vi "430_RS232_Query.vi"(8 "error in (no error)":errorcluster, 9 "Timeout":i32=1000, 10 "Command":string, 11 "VISA resource name":refnum<visa-resource-name>="COM1") -> (0 "error out":errorcluster, 1 "Bytes Read":i32, 2 "Response":string, 3 "VISA resource name out":refnum<visa-resource-name>="COM1", 4 "Bytes Written":i32)   [LabVIEW 2017]
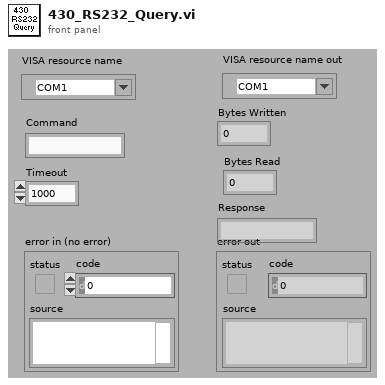
[diagram p1: front panel]
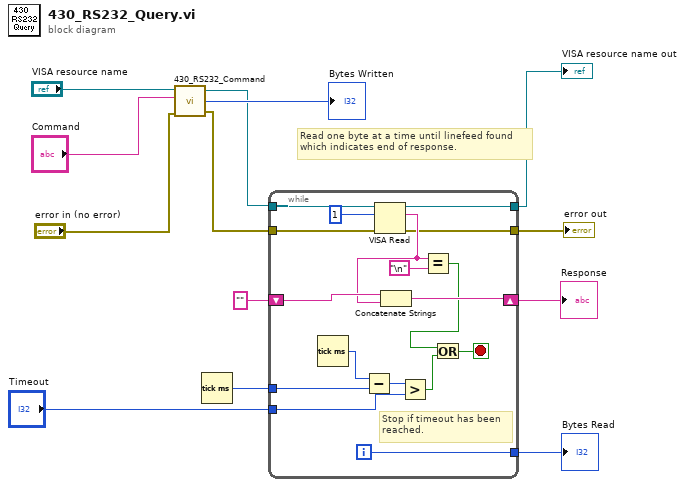
[diagram p0: block diagram]
diagram:
  # "Read one byte at a time until linefeed found\nwhich indicates end of response."
  n1 = call "430_RS232_Command.vi"("error in (no error)"="error in (no error)", "Command"="Command", "VISA resource name"="VISA resource name") -> ("error out"=w7:errorcluster, "bytes written"=→"Bytes Written":i32, "VISA resource name out"=w3:refnum<visa-resource-name>)  [unwired: 1 in]
  n2 = Tick Count (ms)() -> (millisecond timer value=w9:u32)
  n3 = while {
    tunnel: w3 -> [w15]
    tunnel: [w30] -> w4
    tunnel: w7 -> [w29]
    tunnel: [w16] -> w13
    tunnel: [w28] -> w12
    shift-right: [w24] -> w10
    shift-left: "" -> [w26]
    tunnel: "Timeout" -> [w17]
    tunnel: w9 -> [w22]
    i -> [w28]
    stop <- w18 stop-if-true
    # "Stop if timeout has been\nreached."
    n4 = Tick Count (ms)() -> (millisecond timer value=w23:u32)
    n5 = Subtract(x=w23, y=w22) -> (x-y=w21:u32)
    n6 = VISA Read(VISA resource name=w15, byte count=1 ("bytes to read"), error in (no error)=w29) -> (VISA resource name out=w30:refnum<visa-resource-name>, read buffer=w25:string, error out=w16:errorcluster)  [unwired: 1 out]
    n7 = Concatenate Strings(w26, w25) -> (w24:string)
    n8 = Greater?(x=w21, y=w17) -> (0:w20:bool)
    n9 = Equal?(x=w25, y="\n") -> (x = y?=w19:bool)
    n10 = Or(x=w19, y=w20) -> (x .or. y?=w18:bool)
  }
  "error out" <- w13
  "Bytes Read" <- w12
  "Response" <- w10
  "VISA resource name out" <- w4
